vi "Create.vi"(8 "error in (no error)":errorcluster) -> (0 "error out":errorcluster, 3 "IsRefnum":refnum<class "IsRefnum.lvclass">)   [LabVIEW 2017, in "Transparent Assertions.lvlib" / "IsRefnum.lvclass"]
uses:
  IsRefnum.lvclass
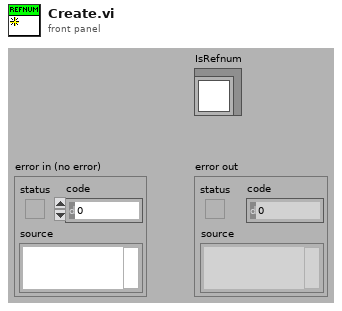
[diagram p1: front panel]
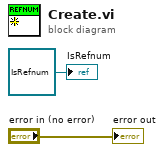
[diagram p0: block diagram]
diagram:
  "error out" <- "error in (no error)"
  "IsRefnum" <- refnum<class "IsRefnum.lvclass"> refnum ("IsRefnum In")
